vi "FRCts20_Backend_SaveXMLData.vi"(6 "Message Attributes":T4, 8 "error in (no error)":errorcluster, 10 "Data":string, 11 "Engine_Refnums":T1) -> (0 "error out":errorcluster)   [LabVIEW 2014, in "FRCts20_Backend_Engine.lvlib"]
doc: "Backs up current xml save, then creates a temp file, stores the cluster, and copies the temp file to the main dir."
uses:
  FRCts20_Backend_Engine.lvlib
  Dependencies/Keyed Array/KeyedArray.ctl
  FRCts20_Backend_EngineRefnums.ctl
  INI_Accessor/FRCts20_Backend_INI Controller.lvclass
  Dependencies/AMC/_SubVIs/TypeDefs/Message Queue.ctl
  Dependencies/AMC/_SubVIs/TypeDefs/Message.ctl
  <vilib>/addons/database/Connection.llb/Conn ObjectReference.ctl
  FRCts20_Backend_FGVOperation.ctl
  FRCts20_Backend_API/FRCts20_Backend_API_Application.ctl
  Dependencies/Keyed Array/Tools_KeyedArray.lvlib
  Dependencies/AMC/AMC.lvlib
  <vilib>/addons/database/NI_Database_API.lvlib
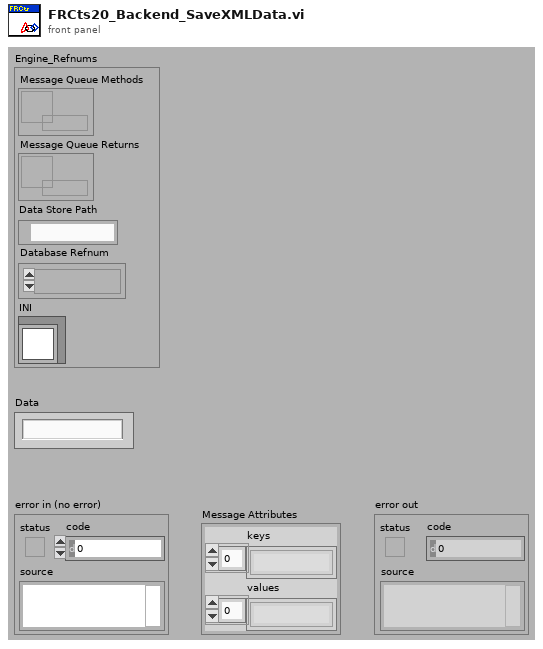
[diagram p1: front panel]
types:
  T1 = typedef "FRCts20_Backend_Engine.lvlib/FRCts20_Backend_EngineRefnums.ctl" = cluster{"Message Queue Methods":T2, "Message Queue Returns":T2, "Data Store Path":path, "Database Refnum":T3, "INI":refnum<class "FRCts20_Backend_INI Controller.lvclass">}
  T2 = typedef "AMC.lvlib/Message Queue.ctl" = refnum<queue>
  T3 = typedef "NI_Database_API.lvlib/Conn ObjectReference.ctl" = refnum<k1>
  T4 = typedef "Tools_KeyedArray.lvlib/KeyedArray.ctl" = cluster{"keys":string[], "values":string[]}
  T5 = enum16{"open", "replace", "create", "open or create", "replace or create", "replace or create with confirmation"}
  T6 = typedef "FRCts20_Backend_API_Application.ctl" = cluster{"Revision":string, "APIReturn":string}
  T7 = typedef "FRCts20_Backend_Engine.lvlib/FRCts20_Backend_FGVOperation.ctl" = enum16{"Initialize", "EnqueueMessage", "EnqueueDataReturn", "FlushMessage", "FlushDataReturn"}
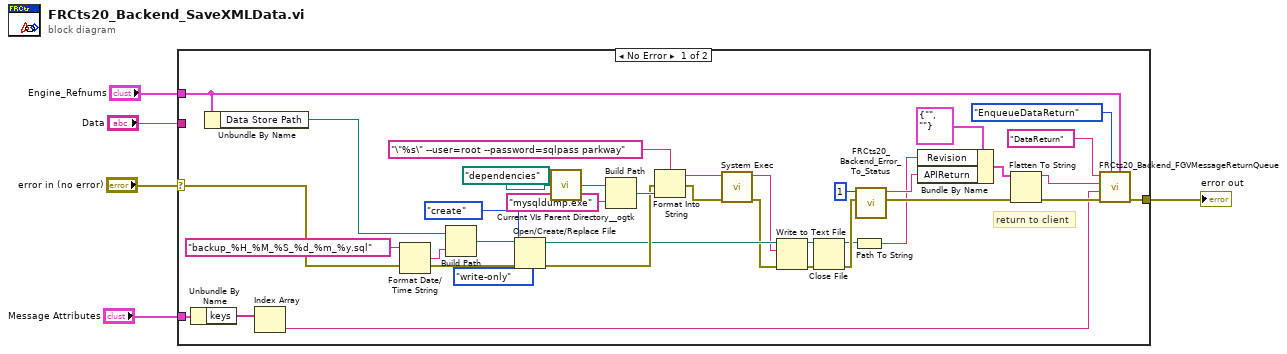
[diagram p0: block diagram]
diagram:
  n1 = case shown="No Error" "error in (no error)" {
    selector: "error in (no error)" -> [w15 w43]
    tunnel: [w32 w43] -> w4
    tunnel: "Engine_Refnums" -> [w20 _]
    tunnel: "Data" -> [_ _]
    tunnel: "Message Attributes" -> [w31 _]
    frame No Error {
      # "return to client"
      n2 = Unbundle By Name(w31) -> ("keys"=w30:string[])
      n3 = Unbundle By Name(w20) -> ("Data Store Path"=w19:path)
      n4 = Index Array(array=w30) -> (element=w29:string)  [unwired: 1 in]
      n5 = Format Date/Time String(time format string (%c)="backup_%H_%M_%S_%d_%m_%y.sql") -> (date/time string=w25:string)  [unwired: 2 in]
      n6 = Build Path(base path=w19, name or relative path=w25) -> (appended path=w18:path)
      n7 = Open/Create/Replace File(file path (use dialog)=w18, error in=w15, operation (0:open)=T5."create", access (0:read/write)=enum16{"read/write", "read-only", "write-only"}."write-only") -> (refnum out=w13:refnum<file>, error out=w14:errorcluster)  [unwired: 2 in, 1 out]
      n8 = call "Current VIs Parent Directory__ogtk.vi"("Relative path (.)"=path "dependencies") -> ("Parent Directory (+ Relative)"=w21:path)  [unwired: 4 in]
      n9 = Build Path(base path=w21, name or relative path="mysqldump.exe") -> (appended path=w23:path)
      n10 = Format Into String(format string="\"%s\" --user=root --password=sqlpass parkway" ("command line"), error in=w14, w23) -> (resulting string=w40:string, error out=w39:errorcluster)  [unwired: 1 in]
      n11 = call <vilib>:"System Exec.vi"("error in (no error)"=w39, "command line"=w40) -> ("error out"=w11:errorcluster, "standard output"=w12:string)  [unwired: 6 in, 2 out]
      n12 = Write to Text File(file (use dialog)=w13, text=w12, error in=w11) -> (refnum out=w9:refnum<file>, error out=w10:errorcluster)  [unwired: 1 in, 1 out]
      n13 = Close File(refnum=w9, error in=w10) -> (path=w7:path, error out=w8:errorcluster)
      n14 = Path To String(path=w7) -> (string=w6:string)
      n15 = call "FRCts20_Backend_Error_To_Status.vi"("error in (no error)"=w8, "rows affected"=1) -> ("error out"=w33:errorcluster, "String"=w26:string)  [unwired: 8 in]
      n16 = Bundle By Name(cluster=T6 {"Revision"="", "APIReturn"=""} ("Application"), "Revision"=w6, "APIReturn"=w26) -> (w27:T6)
      n17 = Flatten To String(anything=w27, error in (no error)=w33) -> (data string=w35:string, error out=w34:errorcluster)  [unwired: 2 in, 1 out]
      n18 = call "FRCts20_Backend_FGVMessageReturnQueue.vi"("Engine_Refnums"=w20, "Operation"=FRCts20_Backend_FGVOperation."EnqueueDataReturn", "error in (no error)"=w34, "Key"=w29, "Message Value"=w35, "Message Name"="DataReturn") -> ("error out"=w32:errorcluster)  [unwired: 4 in, 1 out]
    }
    frame Error {
    }
  }
  "error out" <- w4
